vi "Do.vi"(8 "error in":errorcluster, 10 "Actor in":refnum<class "Actor.lvclass">, 11 "Enable Channel 1 Laser":refnum<class "Update PAS Spk 1 Enable State MSG.lvclass">) -> (0 "error out":errorcluster, 2 "Actor out":refnum<class "Actor.lvclass">)   [LabVIEW 2016, in "Update PAS Spk 1 Enable State MSG.lvclass"]
doc: "(<B>Filename</B>: Actor Framework.lvlib:Message.lvclass:Do.vi)\n\nDefines what a message does when it is received by an actor. Generally, a message instructs an actor to invoke one of its methods. By default, this method does nothing. A child class must override it to define behavior. Create a child class by using the Actor Framework Message Maker dialog box."
uses:
  Update PAS Spk 1 Enable State MSG.lvclass
  gController.lvclass
  <vilib>/rvi/interface/nirviReadWriteControl/nirviReadWriteControl.xnode
  FPGA Ref.ctl
  FPGA Bitfiles/serverv4.lvbitx
  NiFpgaLv.dll
  <vilib>/Utility/error.llb/Error Cluster From Error Code.vi
  <vilib>/rvi/errors/niLvFpgaAdjustHostInterfaceError.vi
  <vilib>/ActorFramework/Actor/Actor.lvclass
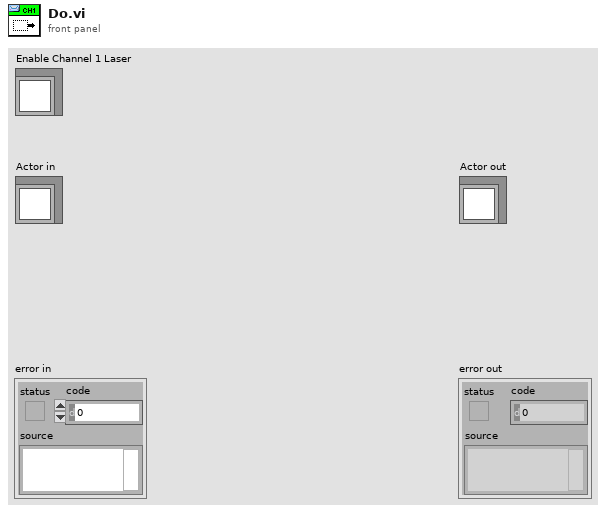
[diagram p1: front panel]
types:
  T1 = typedef "FPGA Ref.ctl" = refnum<k20>
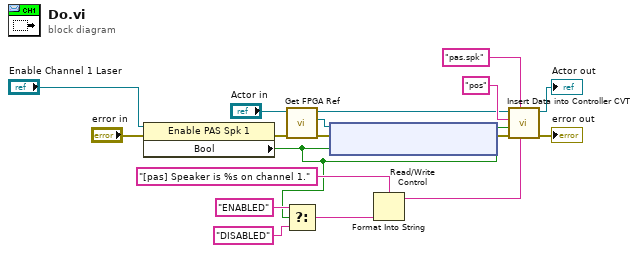
[diagram p0: block diagram]
diagram:
  n1 = property class="Enable PAS Spk 1"(reference="Enable Channel 1 Laser", error in="error in") -> (error out=w5:errorcluster, "Bool"=w1:bool)  [unwired: 1 out]
  n2 = call "Get FPGA Ref.vi"("error in (no error)"=w5, "Actor In"="Actor in") -> ("error out"=w4:errorcluster, "FPGA Ref"=w6:T1, "Actor Out"=w7:refnum<class "Actor.lvclass">)  [unwired: 7 in]
  n3 = Select(t="ENABLED", s=w1, f="DISABLED") -> (s? t:f=w11:string)
  n4 = xnode "Read/Write Control"("FPGA VI Reference In"=w6, "error in"=w4, "spk 1"=w1) -> ("error out"=w3:errorcluster)  [unwired: 1 out]
  n5 = Format Into String(format string="[pas] Speaker is %s on channel 1.", w11) -> (resulting string=w9:string)  [unwired: 2 in, 1 out]
  n6 = call "Insert Data into Controller CVT.vi"("Update MSG"=w9, "Group"="pas.spk", "error in"=w3, "Data"=w1, "tag"="pos", "Actor in"=w7) -> ("error out"=→"error out":errorcluster, "Actor Out"=→"Actor out":refnum<class "Actor.lvclass">)  [unwired: 4 in]
